vi "Salva_comando_Apend.vi"(3 "String":string, 5 "file name p/ exell":string) -> ()   [LabVIEW 2018]
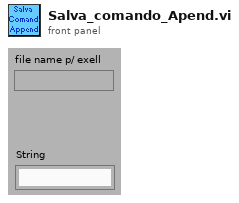
[diagram p1: front panel]
types:
  T1 = enum16{"open", "open or create", "create or replace", "create"}
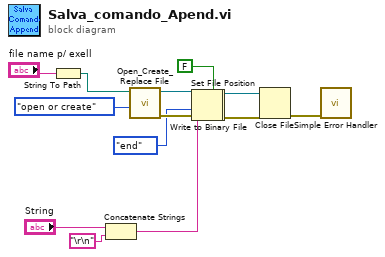
[diagram p0: block diagram]
diagram:
  n1 = String To Path(string="file name p/ exell") -> (path=w8:path)
  n2 = Concatenate Strings("String", "\r\n") -> (w5:string)
  n3 = call <vilib>:"Open_Create_Replace File.vi"("function (open:0)"=T1."open or create", "file path"=w8) -> ("error out"=w11:errorcluster, "refnum"=w14:refnum<file>)  [unwired: 6 in, 2 out]
  n4 = Set File Position(refnum=w14, from (0:start)=enum16{"start", "end", "current"}."end" ("pos mode (0:2)"), error in=w11) -> (refnum out=w3:refnum<file>, error out=w2:errorcluster)  [unwired: 1 in]
  n5 = Write to Binary File(file (use dialog)=w3, data=w5, error in=w2, 5:FALSE ("prepend array or string size? (T)")) -> (refnum out=w13:refnum<file>, error out=w12:errorcluster)  [unwired: 2 in, 1 out]
  n6 = Close File(refnum=w13, error in=w12) -> (error out=w15:errorcluster)  [unwired: 1 out]
  n7 = call <vilib>:"Simple Error Handler.vi"("error in (no error)"=w15) -> ()  [unwired: 4 in, 5 out]
